vi "Defer Panel Updates.vi"(7 "Control":refnum<vi>, 8 "Error In":errorcluster, 11 "Defer Panel Updates":bool) -> (0 "Error Out":errorcluster)   [LabVIEW 2021, in "Seq Edit Quick Drop.lvlib"]
uses:
  Seq Edit Quick Drop.lvlib
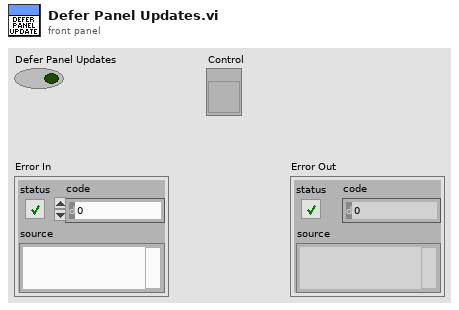
[diagram p1: front panel]
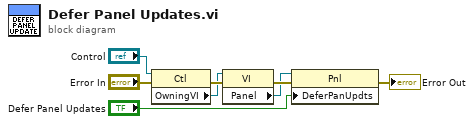
[diagram p0: block diagram]
diagram:
  n1 = property class="Ctl"(reference="Control", error in="Error In") -> (error out=w8:errorcluster, "OwningVI"=w6:refnum<vi>)  [unwired: 1 out]
  n2 = property class="VI"(reference=w6, error in=w8) -> (error out=w7:errorcluster, "Panel"=w5:refnum<vi>)  [unwired: 1 out]
  n3 = property class="Pnl"(reference=w5, error in=w7, "DeferPanUpdts"="Defer Panel Updates") -> (error out=→"Error Out":errorcluster)  [unwired: 1 out]
